vi "QR Code_Initialize.vi"(8 "error in":errorcluster) -> (0 "error out":errorcluster, 3 "Buffer Data":T1)   [LabVIEW 2016]
uses:
  Data Def/QR Code_Buffer Data.ctl
  <vilib>/vision/Image Controls.llb/IMAQ Image.ctl
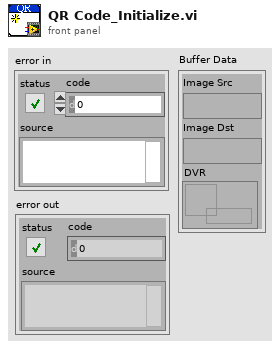
[diagram p1: front panel]
types:
  T1 = typedef "QR Code_Buffer Data.ctl" = cluster{"Image Src":T2, "Image Dst":T2, "DVR":refnum<data-value>}
  T2 = typedef "IMAQ Image.ctl" = refnum<image>
  T3 = typedef "Image Type" = u32
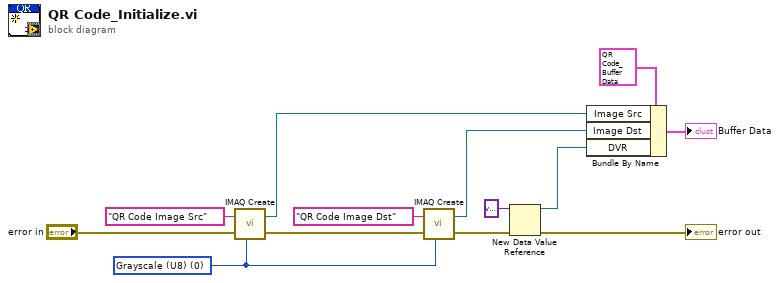
[diagram p0: block diagram]
diagram:
  w1 = T3 0 items=["Grayscale (U8)", "Grayscale (I16)", "Grayscale (SGL)", "Complex (CSG)", "RGB (U32)", "HSL (U32)", "RGB (U64)", "Grayscale (U16)"] ("Image Type")
  n1 = call "IMAQ Create"("Image Name"="QR Code Image Src", "Image Type"=w1, "error in (no error)"="error in") -> ("New Image"=w8:T2, "error out"=w10:errorcluster)  [unwired: 2 in]
  n2 = call "IMAQ Create"("Image Name"="QR Code Image Dst", "Image Type"=w1, "error in (no error)"=w10) -> ("New Image"=w7:T2, "error out"=w4:errorcluster)  [unwired: 2 in]
  n3 = New Data Value Reference(data value=variant, error in=w4) -> (data value reference=w3:refnum<data-value>, error out=→"error out":errorcluster)
  n4 = Bundle By Name(cluster=T1 {"Image Src"=refnum, "Image Dst"=refnum, "DVR"=refnum} ("Buffer Data"), "Image Src"=w8, "Image Dst"=w7, "DVR"=w3) -> (→"Buffer Data":T1)
